vi "ShutdownWindows.vi"() -> ()   [LabVIEW 2018]
panel:
  out "error out":errorcluster
  out "Elapsed Time (s)":dbl
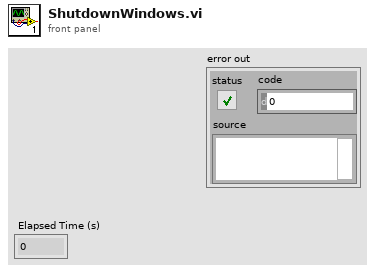
[diagram p1: front panel]
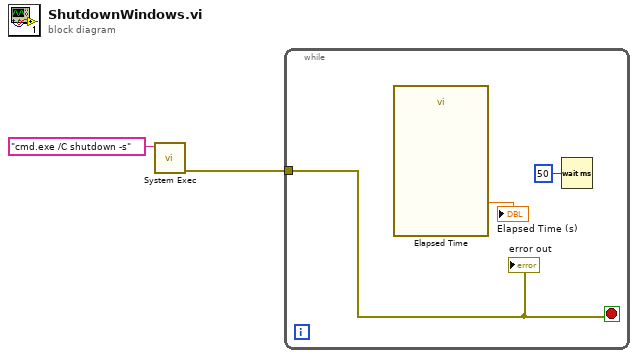
[diagram p0: block diagram]
diagram:
  n1 = call <vilib>:"System Exec.vi"("command line"="cmd.exe /C shutdown -s") -> ("error out"=w1:errorcluster)  [unwired: 7 in, 3 out]
  n2 = while {
    tunnel: w1 -> [w5]
    stop <- w5 stop-if-true
    n3 = call "Elapsed Time"() -> ("Elapsed Time (s)"=→"Elapsed Time (s)":dbl)  [unwired: 12 in, 7 out]
    n4 = Wait (ms)(milliseconds to wait=u32 50) -> ()  [unwired: 1 out]
    "error out" <- w5
  }
